vi "PIM Test Parameters to Stimulus.vi"(10 "PIM Test Parameters":T9={"Stimulus"={"C1 Pwr dBm"=0.0, "C2 Pwr dBm"=0.0, "Power Units"=enum."dBm", "Meas Type"=enum."Time", "C1 Freq MHz"=0.0, "C2 Freq MHz"=0.0, "Swept Freq Step"=0}, "Measure"={"IM Order"=0, "Direction"=0, "Averaging"=1, "ALC ON?"=TRUE, "Peak Hold?"=TRUE, "Peak last N"=1, "Ref Level dBm"=-100.0, "Ref Units"=enum."dBm", "Num Samples"=1, "Sample units"=enum."Sample(s)", "Update Rate (s)"=0.0, "DUT PORT"=enum."Port 1", "Percent (%)"=100}, "Display"={"Power Scale"={"yRange_min"=0, "yRange_max"=0}, "xRange_span"=5}} {"Stimulus"."Swept Freq Step" items=[".2", ".4", "1.0", "2.0"]; "Measure"."Averaging" items=["None", "Minimum", "Normal", "High", "Maximum"]; "Measure"."Direction" items=["Reverse", "Forward", "Auxiliary"]; "Measure"."IM Order" items=["3rd", "5th", "7th", "9th", "11th", "13th", "15th", "17th", "19th", "21st", "23rd", "25th", "27th", "29th", "31st", "33rd"]}) -> (2 "PIM Measurement Stimulus":T1={"Carrier Frequencies"={"C1 Freq, MHz"=0.0, "C2 Freq, MHz"=0.0}, "Carrier Powers"={"C1 Power,dBm"=0.0, "C2 Power, dBm"=0.0}, "Measurement Parameters"={"IM Order"=0, "Averaging"=1, "Direction"=0, "Enable ALC?"=FALSE, "Enable SingleIM?"=FALSE, "Display Units"=enum."dBm", "VA Hold?"=FALSE, "DUT PORT"=enum."Port 1"}, "Measurement Setup"={"Meas Type"=enum."Time", "TXStep"=0}} {"Measurement Setup"."TXStep" items=[".2", ".4", "1.0", "2.0"]; "Measurement Parameters"."Direction" items=["Reverse", "Forward", "Auxiliary"]; "Measurement Parameters"."IM Order" items=["3rd", "5th", "7th", "9th", "11th", "13th", "15th", "17th", "19th", "21st", "23rd", "25th", "27th", "29th", "31st", "33rd"]; "Measurement Parameters"."Averaging" items=["None", "Minimum", "Normal", "High", "Maximum"]})   [LabVIEW 2011]
uses:
  TypeDefs/PIM Test Parameters.ctl
  TypeDefs/PIM Stimulus Parameters.ctl
  BPIMCore/HW IO/PIM Sweep Step Size.ctl
  TypeDefs/PIM Measurement Parameters.ctl
  BPIMCore/HW IO/IMOrder.ctl
  BPIMCore/HW IO/MeasMode.ctl
  BPIMCore/HW IO/HW Averaging.ctl
  TypeDefs/PIM Meas Units.ctl
  BPIMCore/HW IO/DUTport.ctl
  TypeDefs/PIM Display Parameters.ctl
  drivers/PIM/PIM Stimulus.ctl
  drivers/PIM/PIM Cmd Params.ctl
  BPIMCore/Display/display_unit_format.ctl
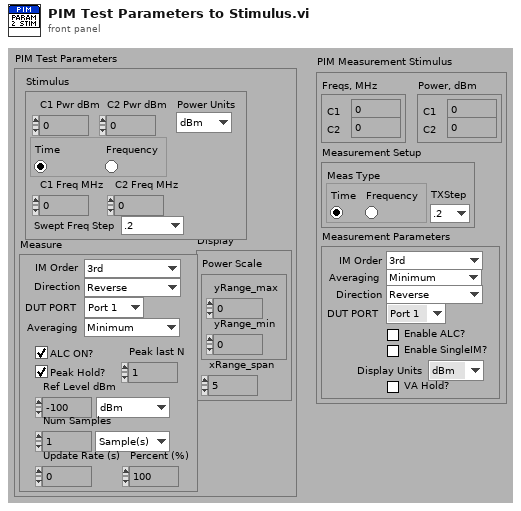
[diagram p1: front panel]
types:
  T1 = typedef "PIM Stimulus.ctl" = cluster{"Carrier Frequencies":cluster{"C1 Freq, MHz":dbl, "C2 Freq, MHz":dbl}, "Carrier Powers":cluster{"C1 Power,dBm":dbl, "C2 Power, dBm":dbl}, "Measurement Parameters":T2, "Measurement Setup":cluster{"Meas Type":enum32{"Time", "Frequency"}, "TXStep":T8}}
  T2 = typedef "PIM Cmd Params.ctl" = cluster{"IM Order":T3, "Averaging":T4, "Direction":T5, "Enable ALC?":bool, "Enable SingleIM?":bool, "Display Units":T6, "VA Hold?":bool, "DUT PORT":T7}
  T3 = typedef "IMOrder.ctl" = u8
  T4 = typedef "HW Averaging.ctl" = u16
  T5 = typedef "MeasMode.ctl" = u16
  T6 = typedef "display_unit_format.ctl" = enum16{"dBm", "dBc"}
  T7 = typedef "DUTport.ctl" = enum16{"Port 1", "Port 2"}
  T8 = typedef "PIM Sweep Step Size.ctl" = u16
  T9 = typedef "PIM Test Parameters.ctl" = cluster{"Stimulus":T10, "Measure":T11, "Display":T13}
  T10 = typedef "PIM Stimulus Parameters.ctl" = cluster{"C1 Pwr dBm":dbl, "C2 Pwr dBm":dbl, "Power Units":enum16{"dBm", "Watts"}, "Meas Type":enum32{"Time", "Frequency"}, "C1 Freq MHz":dbl, "C2 Freq MHz":dbl, "Swept Freq Step":T8}
  T11 = typedef "PIM Measurement Parameters.ctl" = cluster{"IM Order":T3, "Direction":T5, "Averaging":T4, "ALC ON?":bool, "Peak Hold?":bool, "Peak last N":u32, "Ref Level dBm":dbl, "Ref Units":enum16{"dBm", "dBc"}, "Num Samples":u32, "Sample units":T12, "Update Rate (s)":dbl, "DUT PORT":T7, "Percent (%)":u8}
  T12 = typedef "PIM Meas Units.ctl" = enum16{"Sample(s)", "Second(s)", "Sweep(s)"}
  T13 = typedef "PIM Display Parameters.ctl" = cluster{"Power Scale":cluster{"yRange_min":i32, "yRange_max":i32}, "xRange_span":u32}
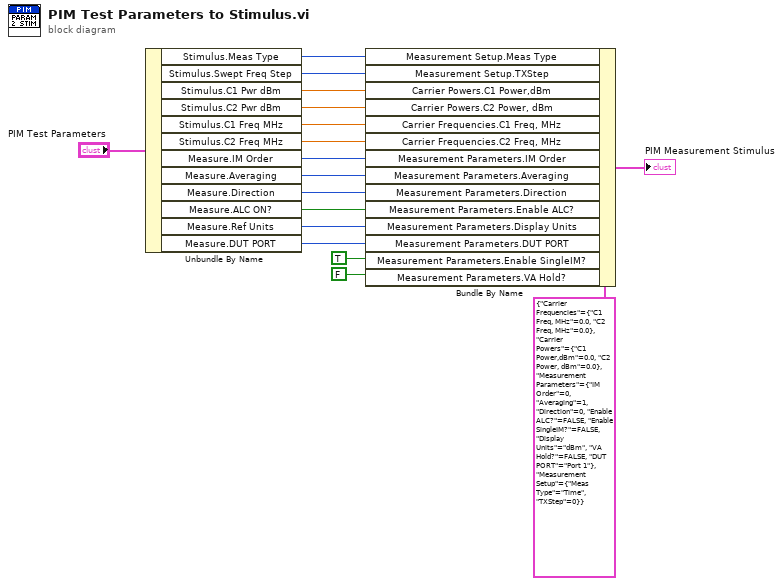
[diagram p0: block diagram]
diagram:
  n1 = Unbundle By Name("PIM Test Parameters") -> ("Stimulus.Meas Type"=w2:enum32{"Time", "Frequency"}, "Stimulus.Swept Freq Step"=w1:T8, "Stimulus.C1 Pwr dBm"=w7:dbl, "Stimulus.C2 Pwr dBm"=w6:dbl, "Stimulus.C1 Freq MHz"=w15:dbl, "Stimulus.C2 Freq MHz"=w14:dbl, "Measure.IM Order"=w13:T3, "Measure.Averaging"=w12:T4, "Measure.Direction"=w11:T5, "Measure.ALC ON?"=w10:bool, "Measure.Ref Units"=w5:enum16{"dBm", "dBc"}, "Measure.DUT PORT"=w3:T7)
  n2 = Bundle By Name(cluster=T1 {"Carrier Frequencies"={"C1 Freq, MHz"=0.0, "C2 Freq, MHz"=0.0}, "Carrier Powers"={"C1 Power,dBm"=0.0, "C2 Power, dBm"=0.0}, "Measurement Parameters"={"IM Order"=0, "Averaging"=1, "Direction"=0, "Enable ALC?"=FALSE, "Enable SingleIM?"=FALSE, "Display Units"=enum."dBm", "VA Hold?"=FALSE, "DUT PORT"=enum."Port 1"}, "Measurement Setup"={"Meas Type"=enum."Time", "TXStep"=0}} ("Stimulus"), "Measurement Setup.Meas Type"=w2, "Measurement Setup.TXStep"=w1, "Carrier Powers.C1 Power,dBm"=w7, "Carrier Powers.C2 Power, dBm"=w6, "Carrier Frequencies.C1 Freq, MHz"=w15, "Carrier Frequencies.C2 Freq, MHz"=w14, "Measurement Parameters.IM Order"=w13, "Measurement Parameters.Averaging"=w12, "Measurement Parameters.Direction"=w11, "Measurement Parameters.Enable ALC?"=w10, "Measurement Parameters.Display Units"=w5, "Measurement Parameters.DUT PORT"=w3, "Measurement Parameters.Enable SingleIM?"=TRUE, "Measurement Parameters.VA Hold?"=FALSE ("Measurement Parameters.Enable SingleIM?")) -> (→"PIM Measurement Stimulus":T1)
